vi "Filter Disconnected Targets.vi"(8 "error in (no error)":errorcluster, 11 "Target List Ref":refnum<vi>) -> (0 "error out":errorcluster)   [LabVIEW 2020]
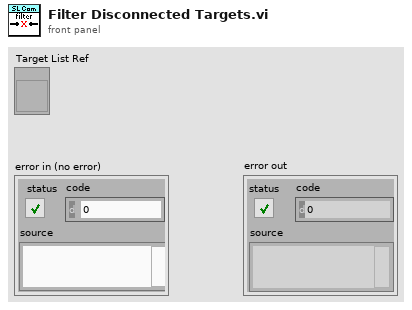
[diagram p1: front panel]
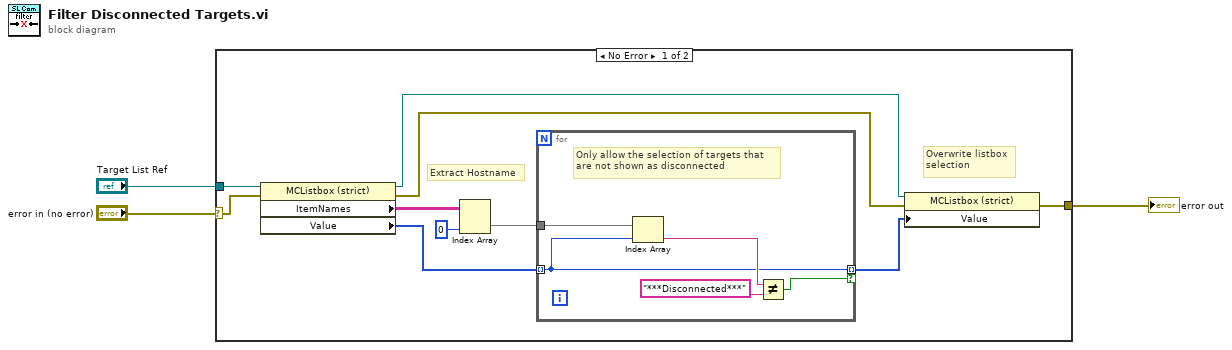
[diagram p0: block diagram]
diagram:
  n1 = case shown="No Error" "error in (no error)" {
    selector: "error in (no error)" -> [w5 w19]
    tunnel: "Target List Ref" -> [w13 _]
    tunnel: [w4 w19] -> w1
    frame No Error {
      # "Overwrite listbox\nselection"
      # "Extract Hostname"
      n2 = property class="MCListbox (strict)"(reference=w13, error in=w5) -> (reference out=w8:refnum<vi>, error out=w7:errorcluster, "ItemNames"=w11:string[][], "Value"=w12:i32[])
      n3 = Index Array "Index Array"(array=w11, index (col)=0 ("disabled index (col)")) -> (element=w9:string[])  [unwired: 1 in]
      n4 = for {
        tunnel: w9 -> [w18]
        tunnel: w12 -> [w15] mode=indexing
        tunnel: [w15] -> w6 mode=indexing if=w14
        # "Only allow the selection of targets that\nare not shown as disconnected"
        n5 = Index Array "Index Array"(array=w18, index=w15) -> (element=w17:string)
        n6 = Not Equal?(x=w17, y="***Disconnected***") -> (x != y?=w14:bool)
      }
      n7 = property class="MCListbox (strict)"(reference=w8, error in=w7, "Value"=w6) -> (error out=w4:errorcluster)  [unwired: 1 out]
    }
    frame Error {
    }
  }
  "error out" <- w1
